vi "build-filepath.vi"(8 "Include Seconds in Filename":bool, 9 "increment file-number":u32=1, 10 "increment filename?":bool, 11 "Log Filepath Selection":T1={"Log Filepath Source"=enum."Application Relative (Auto)", "Log File Path (Manual)"=path "C:/Users/dheard/Documents/0002-labview-projects/ammonia-absorbsion-rig/data", "Log File Folder Name"="data", "log file name"="log", "Include Date in Filename"=TRUE, "Include Time in Filename"=TRUE}) -> (3 "appended path for log file":path, 5 "date string":string)   [LabVIEW 2024]
uses:
  filepath-selection.ctl
panel:
  out "Application Directory":path
  out "datetime-mode":u32
  out "log folder path":path
  out "stripped path":path
  out "vi path":path
  # "Filepath"
  # "File Name"
  # "Auto Generation"
  # "Path is relative to application or VI"
  # "Path Stripped to Local Directory"
  # "This will be the path log files are saved to"
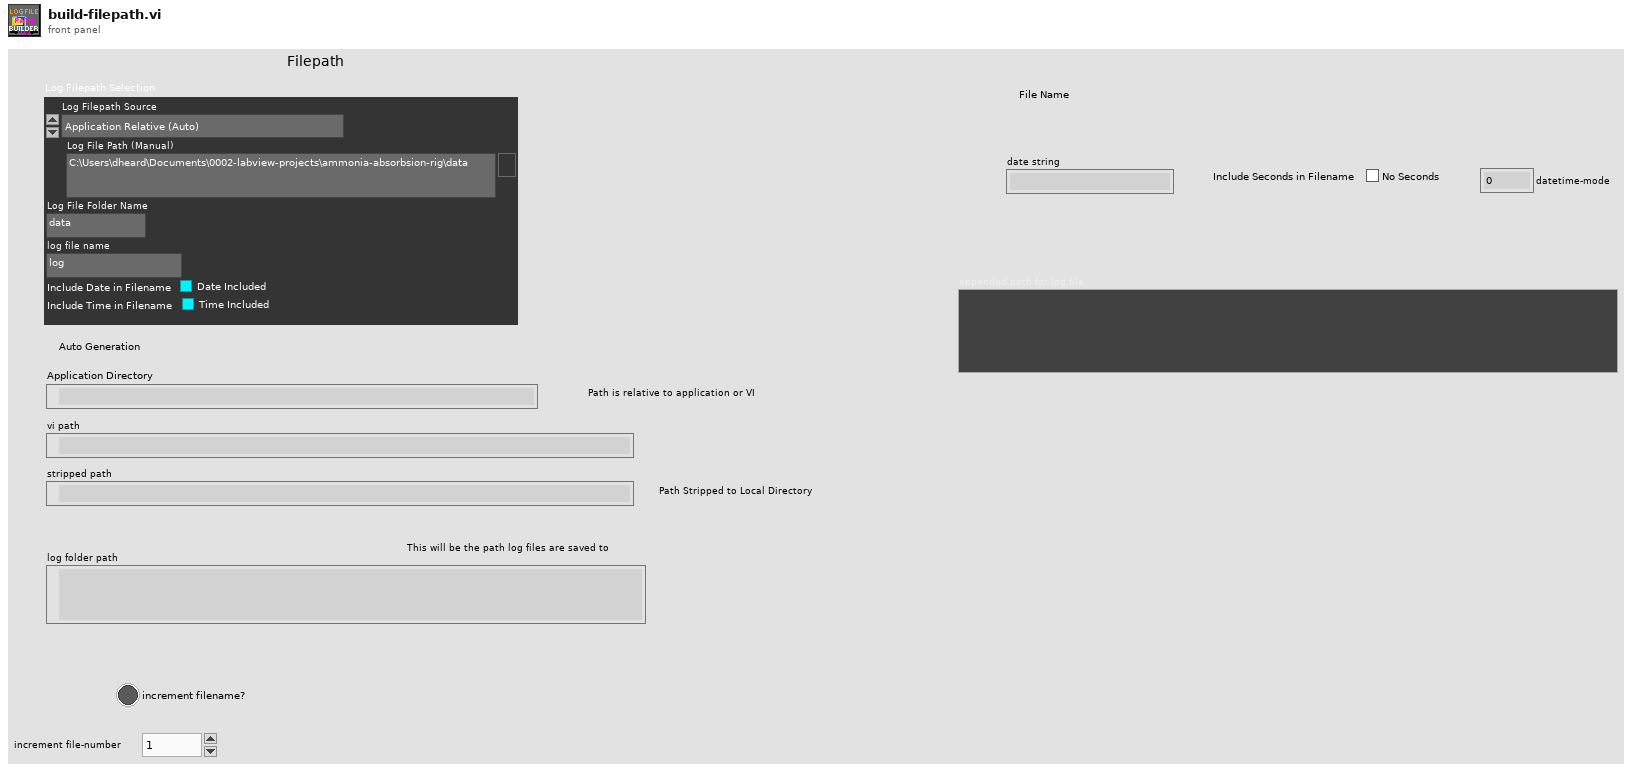
[diagram p1: front panel]
types:
  T1 = typedef "filepath-selection.ctl" = cluster{"Log Filepath Source":enum16{"Application Relative (Auto)", "VI Relative (Auto)", "Complete Path (Manual)"}, "Log File Path (Manual)":path, "Log File Folder Name":string, "log file name":string, "Include Date in Filename":bool, "Include Time in Filename":bool}
  T2 = enum16{"Application Relative (Auto)", "VI Relative (Auto)", "Complete Path (Manual)"}
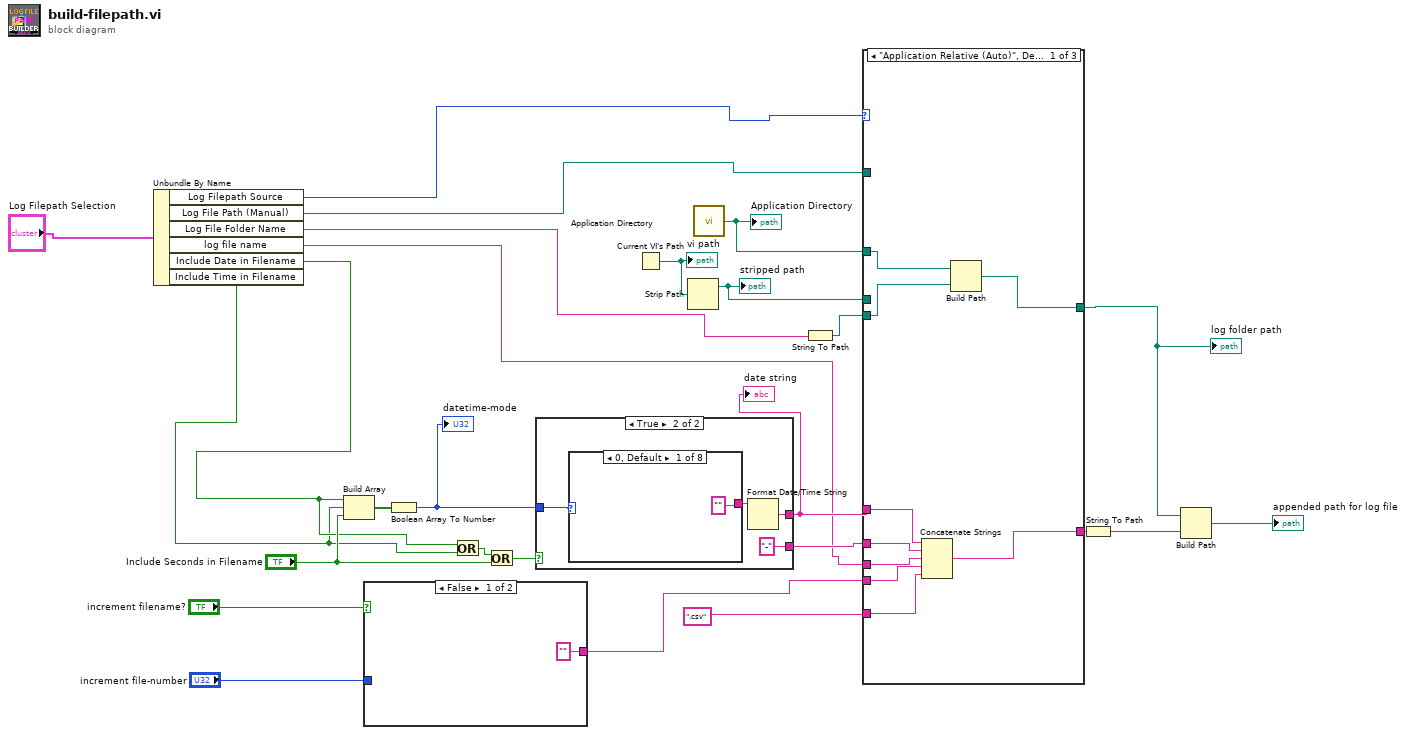
[diagram p0: block diagram]
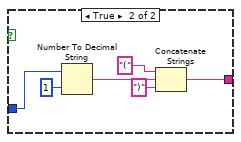
[diagram p2: hidden frame]
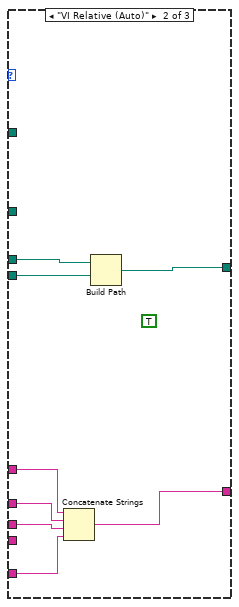
[diagram p3: hidden frame]
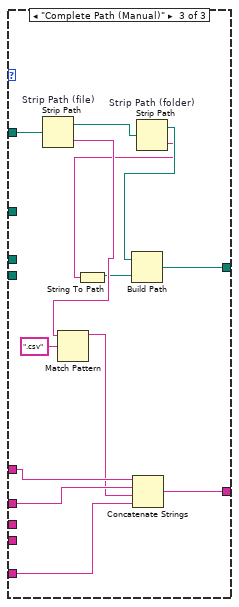
[diagram p4: hidden frame]
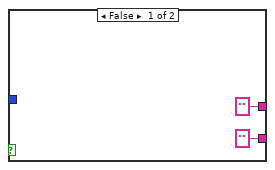
[diagram p5: hidden frame]
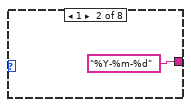
[diagram p6: hidden frame]
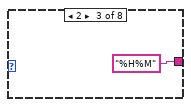
[diagram p7: hidden frame]
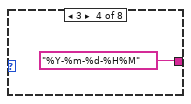
[diagram p8: hidden frame]
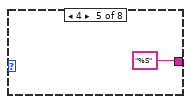
[diagram p9: hidden frame]
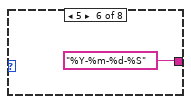
[diagram p10: hidden frame]
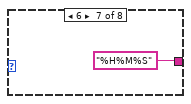
[diagram p11: hidden frame]
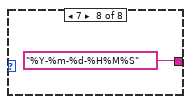
[diagram p12: hidden frame]
diagram:
  n1 = Unbundle By Name("Log Filepath Selection") -> ("Log Filepath Source"=w10:T2, "Log File Path (Manual)"=w9:path, "Log File Folder Name"=w8:string, "log file name"=w5:string, "Include Date in Filename"=w7:bool, "Include Time in Filename"=w6:bool)
  n2 = Build Array(w7, w6, "Include Seconds in Filename") -> (w22:bool[])
  n3 = case shown="False" "increment filename?" {
    tunnel: "increment file-number" -> [_ w33]
    tunnel: ["" w28] -> w1
    frame False {
    }
    frame True {
      n4 = Number To Decimal String(number=w33, width (-)=i16 1) -> (decimal integer string=w31:string)
      n5 = Concatenate Strings("(" ("string"), w31, ")" ("string")) -> (w28:string)
    }
  }
  n6 = Boolean Array To Number(Boolean array=w22) -> (number=w26:u32)
  "datetime-mode" <- w26
  n7 = Or(x=w7, y=w6) -> (x .or. y?=w23:bool)
  n8 = Or(x=w23, y="Include Seconds in Filename") -> (x .or. y?=w24:bool)
  n9 = case shown="True" w24 {
    tunnel: ["" ("date/time string") w39] -> w16
    tunnel: w26 -> [_ w37]
    tunnel: ["" ("string") "-" ("string")] -> w15
    frame False {
    }
    frame True {
      n10 = case shown="0, Default" w37 {
        tunnel: ["" ("time format string (%c)") "%Y-%m-%d" ("time format string (%c)") "%H%M" ("time format string (%c)") "%Y-%m-%d-%H%M" ("time format string (%c)") "%S" ("time format string (%c)") "%Y-%m-%d-%S" ("time format string (%c)") "%H%M%S" ("time format string (%c)") "%Y-%m-%d-%H%M%S" ("time format string (%c)")] -> w38
        frame 0, Default {
        }
        frame 1 {
        }
        frame 2 {
        }
        frame 3 {
        }
        frame 4 {
        }
        frame 5 {
        }
        frame 6 {
        }
        frame 7 {
        }
      }
      n11 = Format Date/Time String(time format string (%c)=w38) -> (date/time string=w39:string)  [unwired: 2 in]
    }
  }
  "date string" <- w16
  n12 = Current VI's Path() -> (path=w19:path)
  "vi path" <- w19
  n13 = Strip Path(path=w19) -> (stripped path=w18:path)  [unwired: 1 out]
  "stripped path" <- w18
  n14 = call <vilib>:"Application Directory.vi"() -> ("Application Directory"=w17:path)
  "Application Directory" <- w17
  n15 = String To Path(string=w8) -> (path=w11:path)
  n16 = case shown="\"Application Relative (Auto)\", Default" w10 {
    tunnel: w18 -> [_ w59 _]
    tunnel: w17 -> [w52 _ _]
    tunnel: w9 -> [_ _ w73]
    tunnel: w16 -> [w54 w63 w75]
    tunnel: w15 -> [w55 w62 w77]
    tunnel: w5 -> [w56 w61 _]
    tunnel: ".csv" ("string") -> [w49 w60 w74]
    tunnel: [w53 w64 w76] -> w13
    tunnel: [w51 w58 w72] -> w12
    tunnel: w11 -> [w50 w57 _]
    tunnel: w1 -> [w48 _ _]
    frame "Application Relative (Auto)", Default {
      n17 = Concatenate Strings(w54, w55, w56, w48, w49) -> (w53:string)
      n18 = Build Path(base path=w52, name or relative path=w50) -> (appended path=w51:path)
    }
    frame "VI Relative (Auto)" {
      (unwired) TRUE
      n19 = Concatenate Strings(w63, w62, w61, w60) -> (w64:string)
      n20 = Build Path(base path=w59, name or relative path=w57) -> (appended path=w58:path)
    }
    frame "Complete Path (Manual)" {
      n21 = Strip Path "Strip Path (file)"(path=w73) -> (stripped path=w68:path, name=w71:string)
      n22 = Match Pattern(string=w71, regular expression=".csv") -> (before substring=w69:string)  [unwired: 1 in, 3 out]
      n23 = Concatenate Strings(w75, w77, w69, w74) -> (w76:string)
      n24 = Strip Path "Strip Path (folder)"(path=w68) -> (stripped path=w67:path, name=w65:string)
      n25 = String To Path(string=w65) -> (path=w66:path)
      n26 = Build Path(base path=w67, name or relative path=w66) -> (appended path=w72:path)
    }
  }
  "log folder path" <- w12
  n27 = String To Path(string=w13) -> (path=w21:path)
  n28 = Build Path(base path=w12, name or relative path=w21) -> (appended path=→"appended path for log file":path)
